vi "ND_ArrayToNode(viaString).vi"(0 "Tree DVR in":refnum<data-value>, 1 "DBL Array":dbl[](array[numeric]), 3 "error in (no error)":errorcluster, 4 "NodePath":string) -> (7 "error out":errorcluster)   [LabVIEW 2014]
uses:
  <vilib>/MDSplus/Classes/Tree_Class/Tree.lvclass
  <vilib>/MDSplus/Library/MDSplus.lvlib
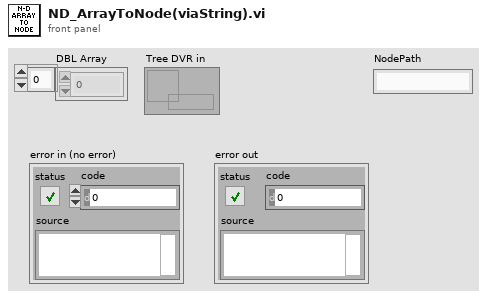
[diagram p1: front panel]
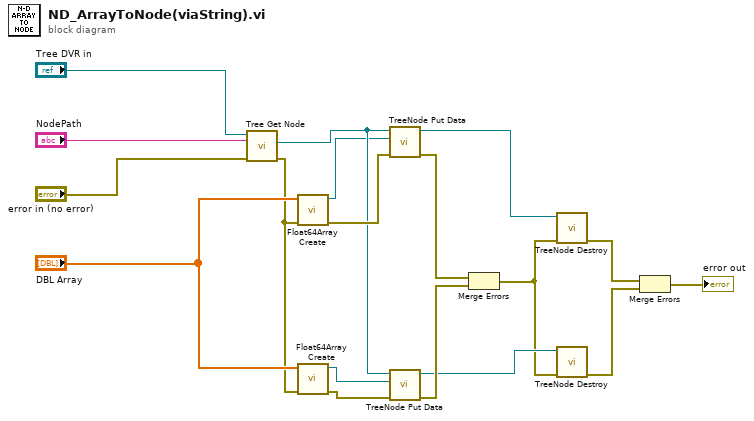
[diagram p0: block diagram]
diagram:
  n1 = call <vilib>:"Tree Get Node.vi"("error in (no error)"="error in (no error)", "Path"="NodePath", "Tree DVR in"="Tree DVR in") -> ("error out"=w13:errorcluster, "Node out"=w9:refnum<data-value>)  [unwired: 6 in, 1 out]
  n2 = call <vilib>:"Float64Array Create.vi"("error in (no error)"=w13, "DBL array in"="DBL Array") -> ("error out"=w15:errorcluster, "Float64Array DVR out"=w7:refnum<data-value>)  [unwired: 8 in]
  n3 = call <vilib>:"Float64Array Create.vi"("error in (no error)"=w13, "DBL array in"="DBL Array") -> ("error out"=w12:errorcluster, "Float64Array DVR out"=w8:refnum<data-value>)  [unwired: 8 in]
  n4 = call <vilib>:"TreeNode Put Data.vi"("error in (no error)"=w15, "Data"=w7, "TreeNode DVR in"=w9) -> ("error out"=w10:errorcluster, "TreeNode DVR out"=w6:refnum<data-value>)  [unwired: 7 in]
  n5 = call <vilib>:"TreeNode Put Data.vi"("error in (no error)"=w12, "Data"=w8, "TreeNode DVR in"=w9) -> ("error out"=w11:errorcluster, "TreeNode DVR out"=w5:refnum<data-value>)  [unwired: 7 in]
  n6 = Merge Errors(w10, w11) -> (w4:errorcluster)
  n7 = call <vilib>:"TreeNode Destroy.vi"("error in (no error)"=w4, "TreeNode DVR in"=w6) -> ("error out"=w2:errorcluster)  [unwired: 9 in]
  n8 = call <vilib>:"TreeNode Destroy.vi"("error in (no error)"=w4, "TreeNode DVR in"=w5) -> ("error out"=w3:errorcluster)  [unwired: 9 in]
  n9 = Merge Errors(w2, w3) -> (→"error out":errorcluster)
